vi "ISweep_skeleton.vi"(1 "DMM1 GPIB address":string="17", 2 "DMM2 GPIB address":string="30", 3 "Main Temperature Controller GPIB address":string="10", 6 "Current rise time (ms)":dbl=100.0, 11 "B/I-factor (Gauss/mA)":dbl format="%.2f", 12 "Setpoint temperature (K)":dbl=22.0 format="%.3f", 14 "File Name":string="IVdata_FeAs_29IV1-2_090311_Rl_2_(0.00Gauss22.000K).txt", 15 "File Path":path=path "c:/data", 16 "Voltage resolution (nV)":dbl=0.5 format="%.1f", 18 "Allowable temperature deviation (K)":dbl=0.002 format="%.4f", 19 "Number of voltage measurements\nbetween temperature check":dbl=8.0) -> ()   [LabVIEW 2014]
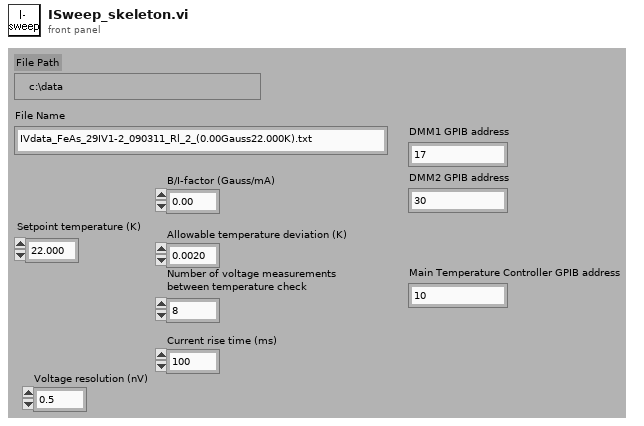
[diagram p1: front panel]
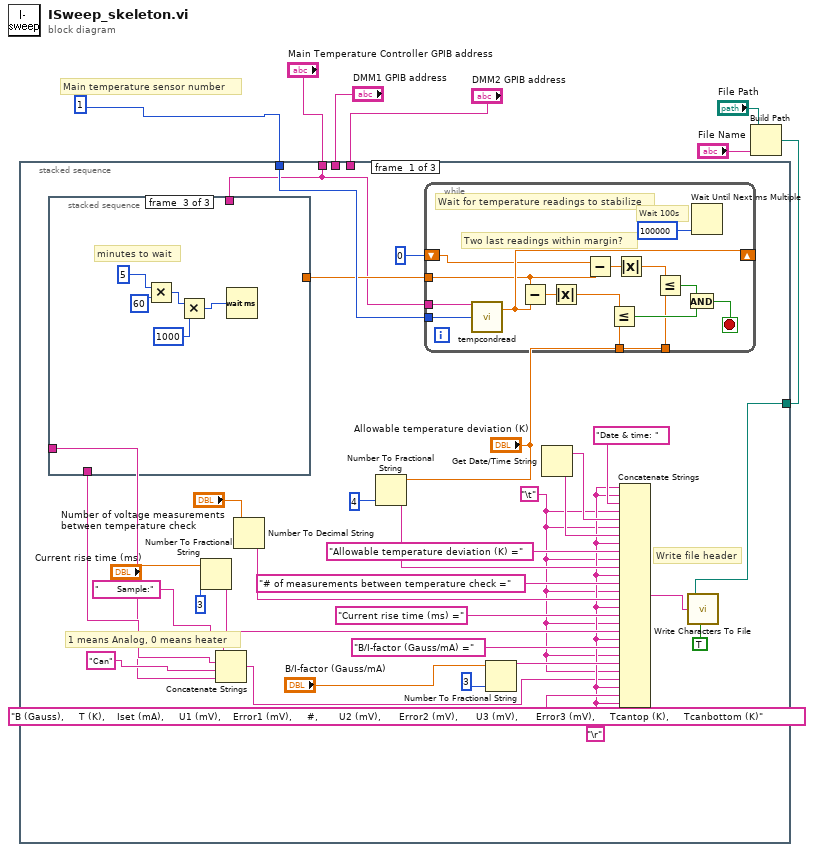
[diagram p0: block diagram]
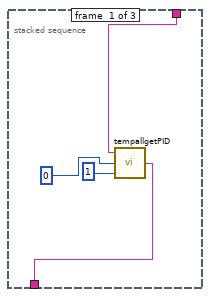
[diagram p2: hidden frame]
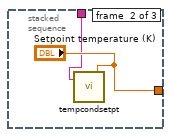
[diagram p3: hidden frame]
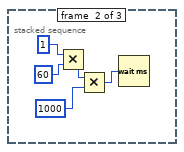
[diagram p4: hidden frame]
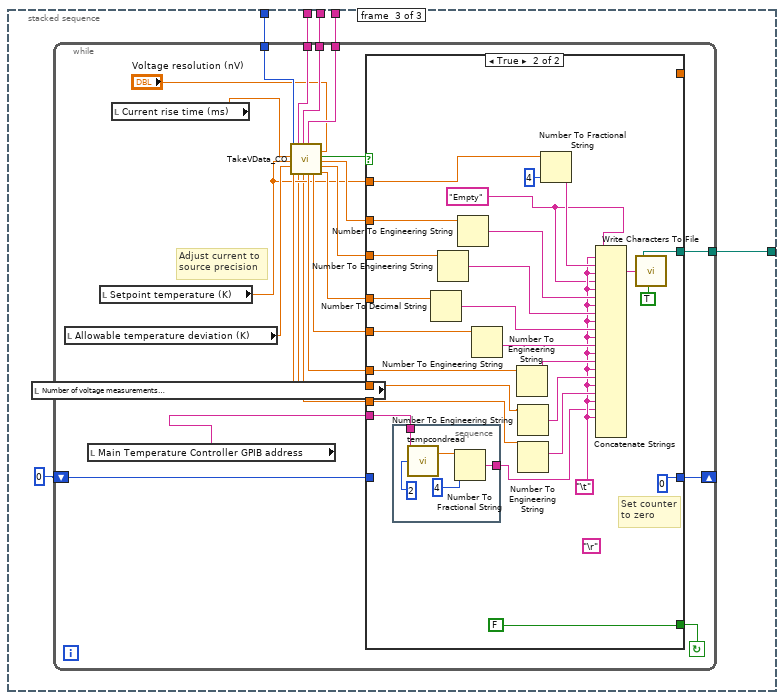
[diagram p5: hidden frame]
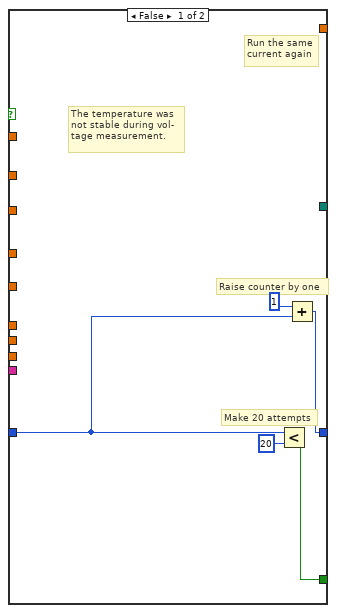
[diagram p6: hidden frame]
diagram:
  # "Main temperature sensor number"
  n1 = Build Path(base path="File Path", name or relative path="File Name") -> (appended path=w7:path)
  n2 = stacked-sequence {
    tunnel: w7 -> [w27 _ w74]
    tunnel: "DMM1 GPIB address" -> [_ _ w77]
    tunnel: 1 -> [w25 _ w75]
    tunnel: "Main Temperature Controller GPIB address" -> [w14 _ w76]
    tunnel: "DMM2 GPIB address" -> [_ _ w72]
    frame #0 {
      w10 = "\t"
      w15 = "\r"
      # "1 means Analog, 0 means heater"
      # "Write file header"
      n3 = stacked-sequence {
        tunnel: w14 -> [w59 w60 _]
        tunnel: [_ "Setpoint temperature (K)" _] -> w17
        tunnel: [w56 _ _] -> w9
        tunnel: [_ _ _] -> w8
        frame #0 {
          n4 = call "tempallgetPID.vi"("Neocera: Heater or Analog;\nLakeshore: Heater 1 or 2"=1, "Temperature controller"=0, "GPIB address"=w59) -> ("Out"=w56:string)
        }
        frame #1 {
          n5 = call "tempcondsetpt.vi"("Set Point"="Setpoint temperature (K)", "GPIB Address"=w60) -> ()  [unwired: 1 in, 1 out]
        }
        frame #2 {
          # "minutes to wait"
          n6 = Multiply(x=5, y=60) -> (x*y=w64:i32)
          n7 = Multiply(x=w64, y=1000) -> (x*y=w66:i32)
          n8 = Wait (ms)(milliseconds to wait=w66) -> ()  [unwired: 1 out]
        }
      }
      n9 = Number To Fractional String(number="Current rise time (ms)", precision (6)=3) -> (F-format string=w29:string)  [unwired: 2 in]
      n10 = Concatenate Strings("      Sample:", w9, "Can", w8) -> (w11:string)
      n11 = Number To Decimal String(number="Number of voltage measurements\nbetween temperature check") -> (decimal integer string=w35:string)  [unwired: 1 in]
      n12 = Number To Fractional String(number="Allowable temperature deviation (K)", precision (6)=4) -> (F-format string=w37:string)  [unwired: 2 in]
      n13 = while {
        tunnel: w17 -> [w41]
        tunnel: "Allowable temperature deviation (K)" -> [w42]
        tunnel: "Allowable temperature deviation (K)" -> [w43]
        tunnel: w14 -> [w44]
        tunnel: w25 -> [w45]
        shift-left: 0 -> [w46]
        shift-right: [w47] -> _
        stop <- w52 stop-if-true
        # "Two last readings within margin?"
        # "Wait for temperature readings to stabilize"
        # "Wait 100s"
        n14 = call "tempcondread.vi"("Ring"=w45, "GPIB Address"=w44) -> ("Temperature"=w47:dbl)  [unwired: 1 in, 1 out]
        n15 = Subtract(x=w41, y=w47) -> (x-y=w54:dbl)
        n16 = Absolute Value(x=w54) -> (abs(x)=w51:dbl)
        n17 = Subtract(x=w46, y=w41) -> (x-y=w50:dbl)
        n18 = Less Or Equal?(x=w51, y=w43) -> (x <= y?=w53:bool)
        n19 = Absolute Value(x=w50) -> (abs(x)=w49:dbl)
        n20 = Less Or Equal?(x=w49, y=w42) -> (x <= y?=w48:bool)
        n21 = And(x=w48, y=w53) -> (x .and. y?=w52:bool)
        n22 = Wait Until Next ms Multiple(millisecond multiple=100000) -> ()  [unwired: 1 out]
      }
      n23 = Number To Fractional String(number="B/I-factor (Gauss/mA)", precision (6)=3) -> (F-format string=w21:string)  [unwired: 2 in]
      n24 = Get Date/Time String() -> (date string=w32:string, time string=w31:string)  [unwired: 3 in]
      n25 = Concatenate Strings(w15, w15, "Date & time: ", w10, w32, w10, w31, w15, "Allowable temperature deviation (K) =", w10, w37, w15, "# of measurements between temperature check =", w10, w35, w15, "Current rise time (ms) =", w10, w29, w15, "B/I-factor (Gauss/mA) =", w10, w21, w10, w11, w15, "B (Gauss),     T (K),    Iset (mA),     U1 (mV),    Error1 (mV),     #,       U2 (mV),      Error2 (mV),      U3 (mV),      Error3 (mV),     Tcantop (K),     Tcanbottom (K)", w15) -> (w39:string)
      n26 = call <vilib>:"Write Characters To File.vi"("append to file? (new file:F)"=TRUE, "character string"=w39, "file path (dialog if empty)"=w27) -> ()  [unwired: 2 in, 1 out]
    }
    frame #1 {
      n27 = Multiply(x=1, y=60) -> (x*y=w68:i32)
      n28 = Multiply(x=w68, y=1000) -> (x*y=w70:i32)
      n29 = Wait (ms)(milliseconds to wait=w70) -> ()  [unwired: 1 out]
    }
    frame #2 {
      n30 = while {
        tunnel: w72 -> [w95]
        shift-left: 0 -> [w96]
        shift-right: [w97] -> _
        tunnel: w74 -> [w99]
        tunnel: w75 -> [w92]
        tunnel: w76 -> [w93]
        tunnel: w77 -> [w94]
        stop <- w98 continue-if-true
        # "Adjust current to\nsource precision"
        n31 = local read "Number of voltage measurements\nbetween temperature check"() -> (w84:dbl)
        n32 = local read "Allowable temperature deviation (K)"() -> (w85:dbl)
        n33 = local read "Main Temperature Controller GPIB address"() -> (w78:string)
        n34 = local read "Setpoint temperature (K)"() -> (w83:dbl)
        n35 = local read "Current rise time (ms)"() -> (w82:dbl)
        n36 = call "TakeVData_CO.vi"("Sensor"=w92, "Measurement wait time (ms)"=w82, "Setpoint temperature (K)"=w83, "Allowable deviation (K)"=w85, "Number of voltage measurements\nbetween temperature check"=w84, "Temperature Controller GPIB address"=w93, "DMM (to sample) GPIB address"=w94, "DMM2 GPIB address"=w95, "Cutoff (nV)"="Voltage resolution (nV)") -> ("Mean Temp (C)"=w81:dbl, "Temp error (C)"=w80:dbl, "Voltage error 2 (mV)"=w87:dbl, "Mean Voltage 2 (mV)"=w88:dbl, "Temperature stable?"=w91:bool, "Mean Voltage 1 (mV)"=w86:dbl, "Voltage error 1 (mV)"=w90:dbl, "Number of measurements"=w89:dbl)  [unwired: 3 in]
        n37 = case shown="True" w91 {
          tunnel: w99 -> [_ w130]
          tunnel: _ -> [w100 _]
          tunnel: [w104 FALSE] -> w98
          tunnel: [w103 0] -> w97
          tunnel: w96 -> [w101 _]
          tunnel: w83 -> [_ w122]
          tunnel: w86 -> [_ w115]
          tunnel: w90 -> [_ w121]
          tunnel: w89 -> [_ w120]
          tunnel: w88 -> [_ w117]
          tunnel: w87 -> [_ w116]
          tunnel: w78 -> [_ w110]
          tunnel: w81 -> [_ w112]
          tunnel: w80 -> [_ w111]
          frame False {
            # "Raise counter by one"
            # "Run the same\ncurrent again"
            # "The temperature was\nnot stable during vol-\ntage measurement."
            # "Make 20 attempts"
            n38 = Less?(x=w101, y=20) -> (x < y?=w104:bool)
            n39 = Add(x=1, y=w101) -> (x+y=w103:i32)
          }
          frame True {
            w106 = "Empty"
            (unwired) "\r"
            w109 = "\t"
            # "Set counter\nto zero"
            n40 = stacked-sequence {
              tunnel: w110 -> [w133]
              tunnel: [w132] -> w108
              frame #0 {
                n41 = call "tempcondread.vi"("Ring"=2, "GPIB Address"=w133) -> ("Temperature"=w136:dbl)  [unwired: 1 in, 1 out]
                n42 = Number To Fractional String(number=w136, precision (6)=4) -> (F-format string=w132:string)  [unwired: 2 in]
              }
            }
            n43 = Number To Decimal String(number=w120) -> (decimal integer string=w125:string)  [unwired: 1 in]
            n44 = Number To Engineering String(4:w121) -> (0:w128:string)  [unwired: 3 in]
            n45 = Number To Engineering String(4:w115) -> (0:w129:string)  [unwired: 3 in]
            n46 = Number To Engineering String(4:w117) -> (0:w119:string)  [unwired: 3 in]
            n47 = Number To Engineering String(4:w116) -> (0:w118:string)  [unwired: 3 in]
            n48 = Number To Engineering String(4:w112) -> (0:w114:string)  [unwired: 3 in]
            n49 = Number To Engineering String(4:w111) -> (0:w113:string)  [unwired: 3 in]
            n50 = Number To Fractional String(number=w122, precision (6)=4) -> (F-format string=w123:string)  [unwired: 2 in]
            n51 = Concatenate Strings(w106, w109, w123, w109, w106, w109, w129, w109, w128, w109, w125, w109, w119, w109, w118, w109, w114, w109, w113, w109, w108, w109) -> (w127:string)  [unwired: 2 in]
            n52 = call <vilib>:"Write Characters To File.vi"("append to file? (new file:F)"=TRUE, "character string"=w127, "file path (dialog if empty)"=w130) -> ()  [unwired: 2 in, 1 out]
          }
        }
      }
    }
  }
